vi "Generate Regexp and Name List.vi"(10 "Options (Default)":T4, 11 "Part List":T1[](array[typedef])) -> (2 "Name List":string[](array[string]), 3 "Result":string)   [LabVIEW 2020, in "Stream.lvlib" / "URLPattern.lvclass"]
uses:
  URLPattern.lvclass
  Pattern String Options.ctl
  Pattern Part.ctl
  Pattern Part Type.ctl
  Pattern Part Modifier.ctl
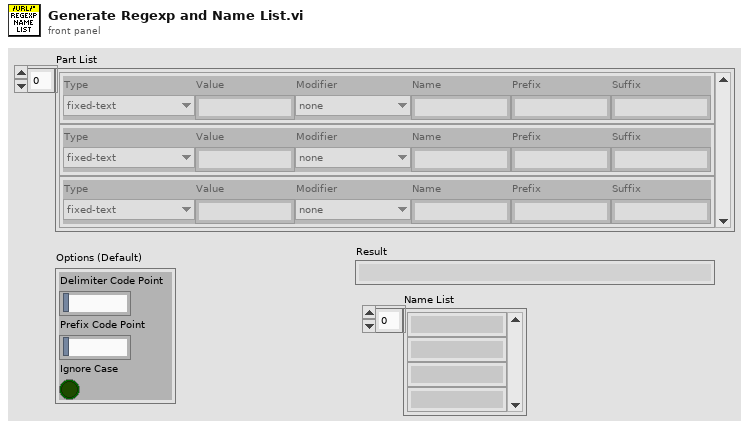
[diagram p1: front panel]
types:
  T1 = typedef "Stream.lvlib/URLPattern.lvclass/Pattern Part.ctl" = cluster{"Type":T2, "Value":string, "Modifier":T3, "Name":string, "Prefix":string, "Suffix":string}
  T2 = typedef "Stream.lvlib/URLPattern.lvclass/Pattern Part Type.ctl" = enum16{"fixed-text", "regexp", "segment-wildcard", "full-wildcard"}
  T3 = typedef "Stream.lvlib/URLPattern.lvclass/Pattern Part Modifier.ctl" = enum16{"none", "optional", "zero-or-more", "one-or-more"}
  T4 = typedef "Stream.lvlib/URLPattern.lvclass/Pattern String Options.ctl" = cluster{"Delimiter Code Point":string, "Prefix Code Point":string, "Ignore Case":bool}
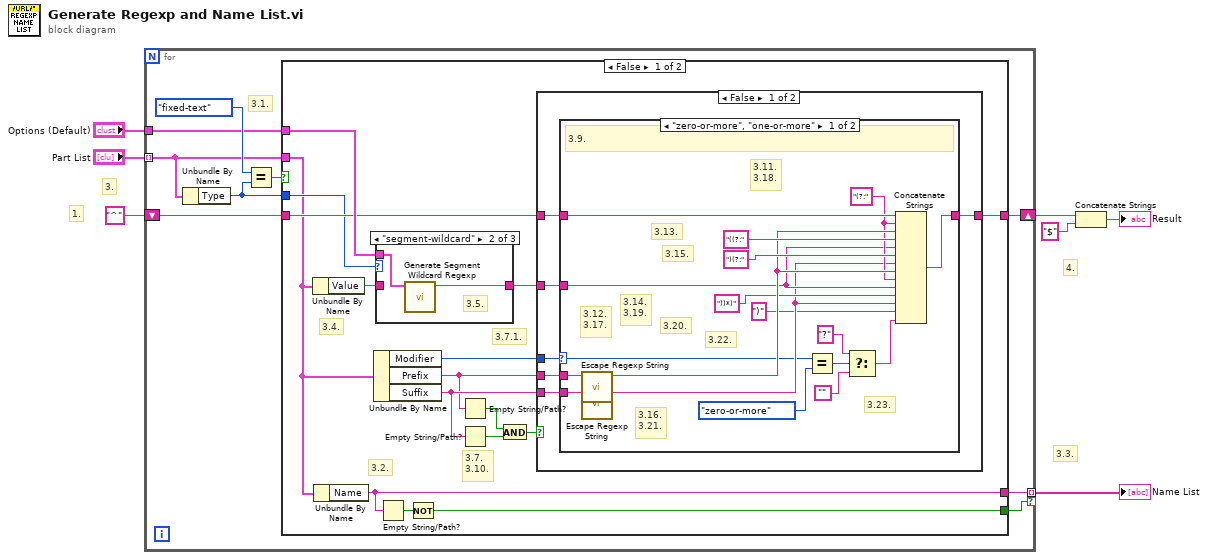
[diagram p0: block diagram]
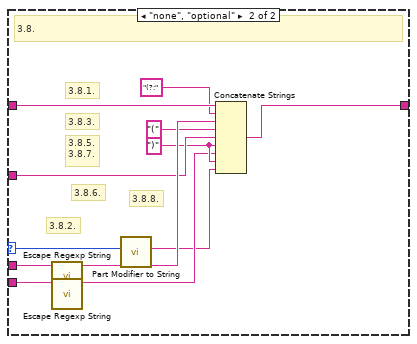
[diagram p2: hidden frame]
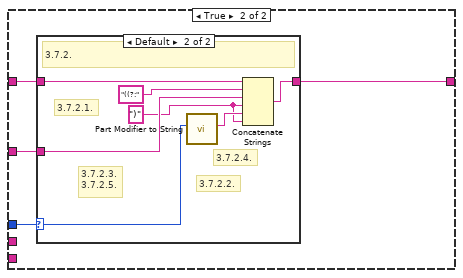
[diagram p3: hidden frame]
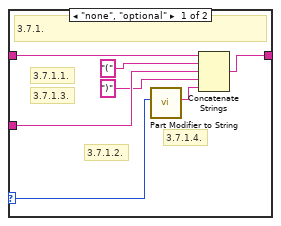
[diagram p4: hidden frame]
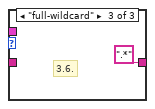
[diagram p6: hidden frame]
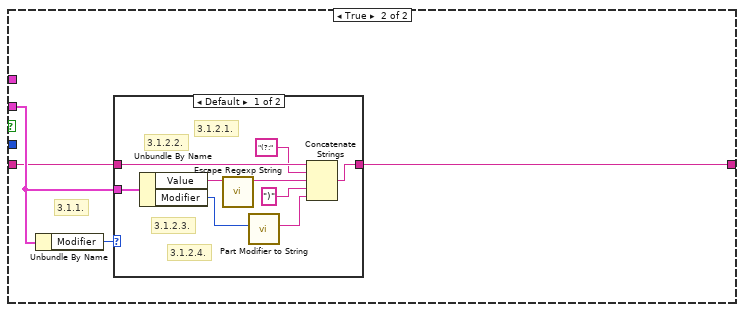
[diagram p7: hidden frame]
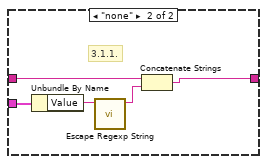
[diagram p8: hidden frame]
diagram:
  # "4."
  # "3.3."
  # "1."
  # "3."
  n1 = for {
    tunnel: "Part List" -> [w13] mode=indexing
    tunnel: "Options (Default)" -> [w12]
    shift-right: [w10] -> w3
    shift-left: "^" -> [w15]
    tunnel: [w9] -> w4 mode=indexing if=w8
    # "3.1."
    n2 = Unbundle By Name(w13) -> ("Type"=w11:T2)
    n3 = Equal?(x=Pattern_Part_Type."fixed-text", y=w11) -> (x = y?=w14:bool)
    n4 = case shown="False" w14 {
      tunnel: w15 -> [w24 w92]
      tunnel: w13 -> [w21 w93]
      tunnel: w12 -> [w32 _]
      tunnel: w11 -> [w23 _]
      tunnel: [w22 w91] -> w10
      tunnel: [w31 _] -> w9
      tunnel: [w25 _] -> w8
      frame False {
        # "3.7.1."
        # "3.7.\n3.10."
        # "3.4."
        # "3.2."
        n5 = Unbundle By Name(w21) -> ("Value"=w30:string)
        n6 = Unbundle By Name(w21) -> ("Name"=w31:string)
        n7 = Unbundle By Name(w21) -> ("Modifier"=w28:T3, "Prefix"=w19:string, "Suffix"=w20:string)
        n8 = case shown="\"segment-wildcard\"" w23 {
          tunnel: w30 -> [w87 _ _]
          tunnel: [w87 w89 ".*" ("Segment Wildcard Regexp")] -> w27
          tunnel: w32 -> [_ w88 _]
          frame Default {
          }
          frame "segment-wildcard" {
            # "3.5."
            n9 = call "Generate Segment Wildcard Regexp.vi"("Options"=w88) -> ("Segment Wildcard Regexp"=w89:string)  [unwired: 10 in]
          }
          frame "full-wildcard" {
            # "3.6."
          }
        }
        n10 = Empty String/Path?(string/path=w31) -> (empty?=w26:bool)
        n11 = Not(x=w26) -> (.not. x?=w25:bool)
        n12 = Empty String/Path?(string/path=w19) -> (empty?=w18:bool)
        n13 = Empty String/Path?(string/path=w20) -> (empty?=w17:bool)
        n14 = And(x=w18, y=w17) -> (x .and. y?=w29:bool)
        n15 = case shown="False" w29 {
          tunnel: w28 -> [w38 w71]
          tunnel: w27 -> [w36 w70]
          tunnel: w24 -> [w37 w72]
          tunnel: [w33 w69] -> w22
          tunnel: w20 -> [w35 _]
          tunnel: w19 -> [w34 _]
          frame False {
            n16 = case shown="\"zero-or-more\", \"one-or-more\"" w38 {
              selector: w38 -> [w45 w59]
              tunnel: w37 -> [w56 w68]
              tunnel: w36 -> [w49 w62]
              tunnel: w35 -> [w54 w67]
              tunnel: w34 -> [w55 w66]
              tunnel: [w39 w57] -> w33
              frame "zero-or-more", "one-or-more" {
                w50 = "(?:" ("string")
                # "3.23."
                # "3.22."
                # "3.20."
                # "3.15."
                # "3.14.\n3.19."
                # "3.13."
                # "3.16.\n3.21."
                # "3.12.\n3.17."
                # "3.11.\n3.18."
                # "3.9."
                n17 = call "Escape Regexp String.vi"("Input"=w55) -> ("Escaped Regexp String"=w51:string)  [unwired: 10 in]
                n18 = call "Escape Regexp String.vi"("Input"=w54) -> ("Escaped Regexp String"=w47:string)  [unwired: 10 in]
                n19 = Equal?(x=w45, y=Pattern_Part_Modifier."zero-or-more") -> (x = y?=w43:bool)
                n20 = Select(t="?", s=w43, f="") -> (s? t:f=w40:string)
                n21 = Concatenate Strings(w56, w50, w51, "((?:" ("string"), w49, ")(?:" ("string"), w47, w51, w50, w49, "))*)" ("string"), w47, ")" ("string"), w40) -> (w39:string)
              }
              frame "none", "optional" {
                w61 = ")" ("string")
                # "3.8.8."
                # "3.8.6."
                # "3.8.5.\n3.8.7."
                # "3.8.3."
                # "3.8.2."
                # "3.8.1."
                # "3.8."
                n22 = call "Escape Regexp String.vi"("Input"=w66) -> ("Escaped Regexp String"=w64:string)  [unwired: 10 in]
                n23 = call "Escape Regexp String.vi"("Input"=w67) -> ("Escaped Regexp String"=w60:string)  [unwired: 10 in]
                n24 = call "Part Modifier to String.vi"("Pattern Part Modifier"=w59) -> ("String"=w58:string)  [unwired: 10 in]
                n25 = Concatenate Strings(w68, "(?:" ("string"), w64, "(" ("string"), w62, w61, w60, w61, w58) -> (w57:string)
              }
            }
          }
          frame True {
            n26 = case shown="Default" w71 {
              selector: w71 -> [w75 w83]
              tunnel: w72 -> [w79 w86]
              tunnel: w70 -> [w77 w84]
              tunnel: [w73 w81] -> w69
              frame "none", "optional" {
                # "3.7.1.4."
                # "3.7.1.3."
                # "3.7.1.2."
                # "3.7.1.1."
                # "3.7.1."
                n27 = call "Part Modifier to String.vi"("Pattern Part Modifier"=w75) -> ("String"=w74:string)  [unwired: 10 in]
                n28 = Concatenate Strings(w79, "(" ("string"), w77, ")" ("string"), w74) -> (w73:string)
              }
              frame Default {
                w80 = ")" ("string")
                # "3.7.2.4."
                # "3.7.2.3.\n3.7.2.5."
                # "3.7.2.2."
                # "3.7.2.1."
                # "3.7.2."
                n29 = call "Part Modifier to String.vi"("Pattern Part Modifier"=w83) -> ("String"=w82:string)  [unwired: 10 in]
                n30 = Concatenate Strings(w86, "((?:" ("string"), w84, w80, w82, w80) -> (w81:string)
              }
            }
          }
        }
      }
      frame True {
        # "3.1.1."
        n31 = Unbundle By Name(w93) -> ("Modifier"=w94:T3)
        n32 = case shown="Default" w94 {
          tunnel: w93 -> [w101 w108]
          tunnel: w92 -> [w103 w106]
          tunnel: [w95 w104] -> w91
          frame Default {
            # "3.1.2.4."
            # "3.1.2.3."
            # "3.1.2.2."
            # "3.1.2.1."
            n33 = Unbundle By Name(w101) -> ("Value"=w100:string, "Modifier"=w97:T3)
            n34 = call "Escape Regexp String.vi"("Input"=w100) -> ("Escaped Regexp String"=w99:string)  [unwired: 10 in]
            n35 = call "Part Modifier to String.vi"("Pattern Part Modifier"=w97) -> ("String"=w96:string)  [unwired: 10 in]
            n36 = Concatenate Strings(w103, "(?:" ("string"), w99, ")" ("string"), w96) -> (w95:string)
          }
          frame "none" {
            # "3.1.1."
            n37 = Unbundle By Name(w108) -> ("Value"=w107:string)
            n38 = call "Escape Regexp String.vi"("Input"=w107) -> ("Escaped Regexp String"=w105:string)  [unwired: 10 in]
            n39 = Concatenate Strings(w106, w105) -> (w104:string)
          }
        }
      }
    }
  }
  "Name List" <- w4
  n40 = Concatenate Strings(w3, "$" ("string")) -> (→"Result":string)
